vi "CurlingRobotforSweepFPGA.vi"() -> ()   [LabVIEW 2015]
uses:
  <vilib>/IEDriver/SPIandI2C/FPGA/Library/IP SPI&I2C.lvlib
  <vilib>/eio/EIONode/EIONode.xnode
  <vilib>/rvi/eio/common/nirviEmuTemplateMethod_errors.vi
  <vilib>/Platform/TimedLoop/XDataNode/wakeup.ctl
  <vilib>/Platform/TimedLoop/XDataNode/XDNodeRunTimeDep.lvlib
  <vilib>/Platform/TimedLoop/XDataNode/nitl_modes.ctl
  <vilib>/Platform/TimedLoop/XDataNode/timing_clust.ctl
  <vilib>/Platform/TimedLoop/XDataNode/XDataNode.xnode
  <vilib>/IEDriver/SPIandI2C/FPGA/Private/Initialize Port (I2C).vi
  <vilib>/IEDriver/SPIandI2C/FPGA/Private/IP Port (I2C).vi
  <vilib>/IEDriver/SPIandI2C/FPGA/Private/Configure Port (I2C).vi
  <vilib>/IEDriver/SPIandI2C/FPGA/Private/Arm Port (I2C).vi
  <vilib>/IEDriver/SPIandI2C/FPGA/Private/Write Port (I2C).vi
  <vilib>/IEDriver/SPIandI2C/FPGA/Private/Read Port (I2C).vi
panel:
  out "FPGA_I2C_port0":i32
  out "FPGA_I2C_port2":i32
  in  "I2C Protocol Action 2":T1(ring)=enum."Idle"
  in  "I2C Protocol Input Data 2":u8
  out "Write Done 2":bool
  out "Arm Done 2":bool
  out "I2C Protocol Output Data 2":u8
  out "Read Done 2":bool
  in  "I2C Protocol Configure 2":T2 {"Command (Write & Read)" items=["Write & Read", "Write", "Read"]}
  out "Configure Done 2":bool
  out "Steer_Left":i64=56
  in  "QuadENC2Reset 2":bool
  out "Steer_Right":i64=56
  in  "QuadENC3Reset 5":bool
  out "Steer_Rear":i64=56
  in  "QuadENC3Reset 4":bool
  in  "Steer_enable":fxp<+/-,20,5>
  in  "Drive_enable":fxp<+/-,20,5>
  in  "Elmo6_Steer_Rear":fxp<+/-,20,5>
  in  "Elmo5_Steer_Right":fxp<+/-,20,5>
  in  "Elmo4_Steer_Left":fxp<+/-,20,5>
  out "Driving_Rear":i64=56
  in  "QuadENC3Reset 3":bool
  in  "stop 2":bool
  in  "Elmo1_Left":fxp<+/-,20,5>
  in  "Elmo2_Right":fxp<+/-,20,5>
  in  "Elmo3_Rear":fxp<+/-,20,5>
  in  "stop":bool
  out "Driving_Left":i64=56
  in  "QuadENC2Reset":bool
  out "Driving_Right":i64=56
  in  "QuadENC3Reset 2":bool
  in  "I2C Protocol Action 0":T1(ring)=enum."Idle"
  in  "I2C Protocol Input Data 0":u8
  out "Write Done":bool
  out "Arm Done":bool
  out "I2C Protocol Output Data 0":u8
  out "Read Done":bool
  in  "I2C Protocol Configure 0":T2 {"Command (Write & Read)" items=["Write & Read", "Write", "Read"]}
  out "Configure Done":bool
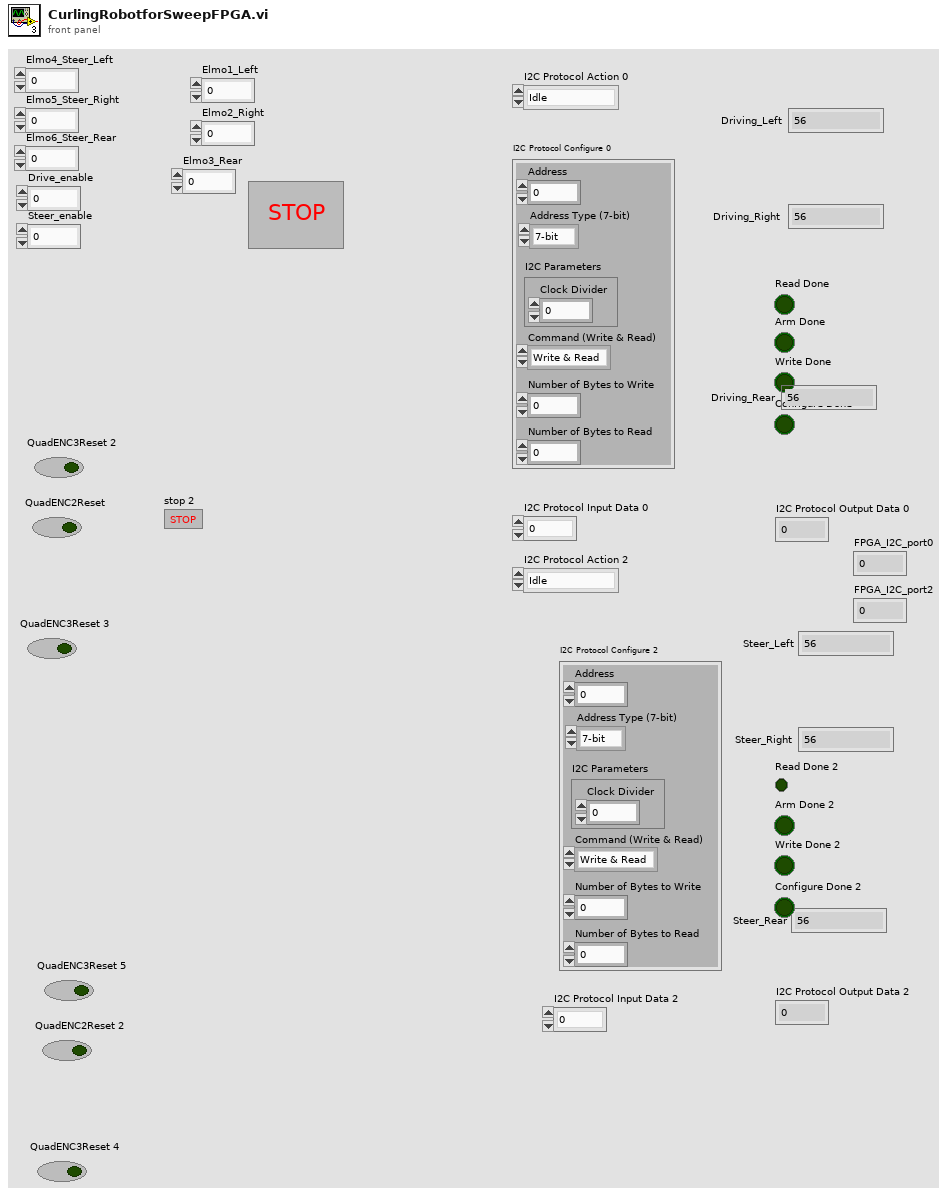
[diagram p1: front panel]
types:
  T1 = enum8{"Configure", "Write", "Arm", "Read", "Set Idle", "Idle"}
  T2 = cluster{"Address":u16, "Address Type (7-bit)":enum16{"7-bit", "10-bit"}, "I2C Parameters":cluster{"Clock Divider":u32}, "Command (Write & Read)":u8, "Number of Bytes to Write":u16, "Number of Bytes to Read":u16}
  T3 = typedef "IP SPI&I2C.lvlib/Private Data (I2C).ctl" = cluster{"Arm Trigger":refnum<k21>, "API to IP Data":refnum<k21>, "IP to API Data":refnum<k21>, "Configuration Register":refnum<k21>, "Configuration Lock":refnum<k21>}
  T4 = typedef "XDNodeRunTimeDep.lvlib/timing_clust.ctl" = cluster{"Expected End [f-1]":u64, "Actual End [f-1]":u64, "Finished Late? [f-1]":bool, "Expected End [i-1]":u64, "Actual End [i-1]":u64, "Finished Late? [i-1]":bool, "Expected Start [i]":u64, "Actual Start [i]":u64, "Expected Start [f]":u64, "Actual Start [f]":u64, "Source Name":string, "Structure Name":string, "Period":i64, "Deadline":i64, "Offset":i64, "Start":i64, "Priority":i32, "Timeout":i32, "Mode":T5, "Wakeup Reason":T6, "Error":errorcluster, "Source Type":string, "Secondary Source Type":string, "Global End Time":u64, "Global Start Time":u64, "Frame Duration":u64, "Iteration Duration":u64, "Assigned CPU":i32, "I/O Scan Engine Mode":u32}
  T5 = typedef "XDNodeRunTimeDep.lvlib/nitl_modes.ctl" = enum32{"No Change", "Process missed periods, maintain original phase", "Discard missed periods, maintain original phase", "Process missed periods, ignore original phase", "Discard missed periods, ignore original phase"}
  T6 = typedef "XDNodeRunTimeDep.lvlib/wakeup.ctl" = enum32{"Normal", "Aborted", "Asynchronous wakeup", "Timing source error", "Timed loop error", "Timeout"}
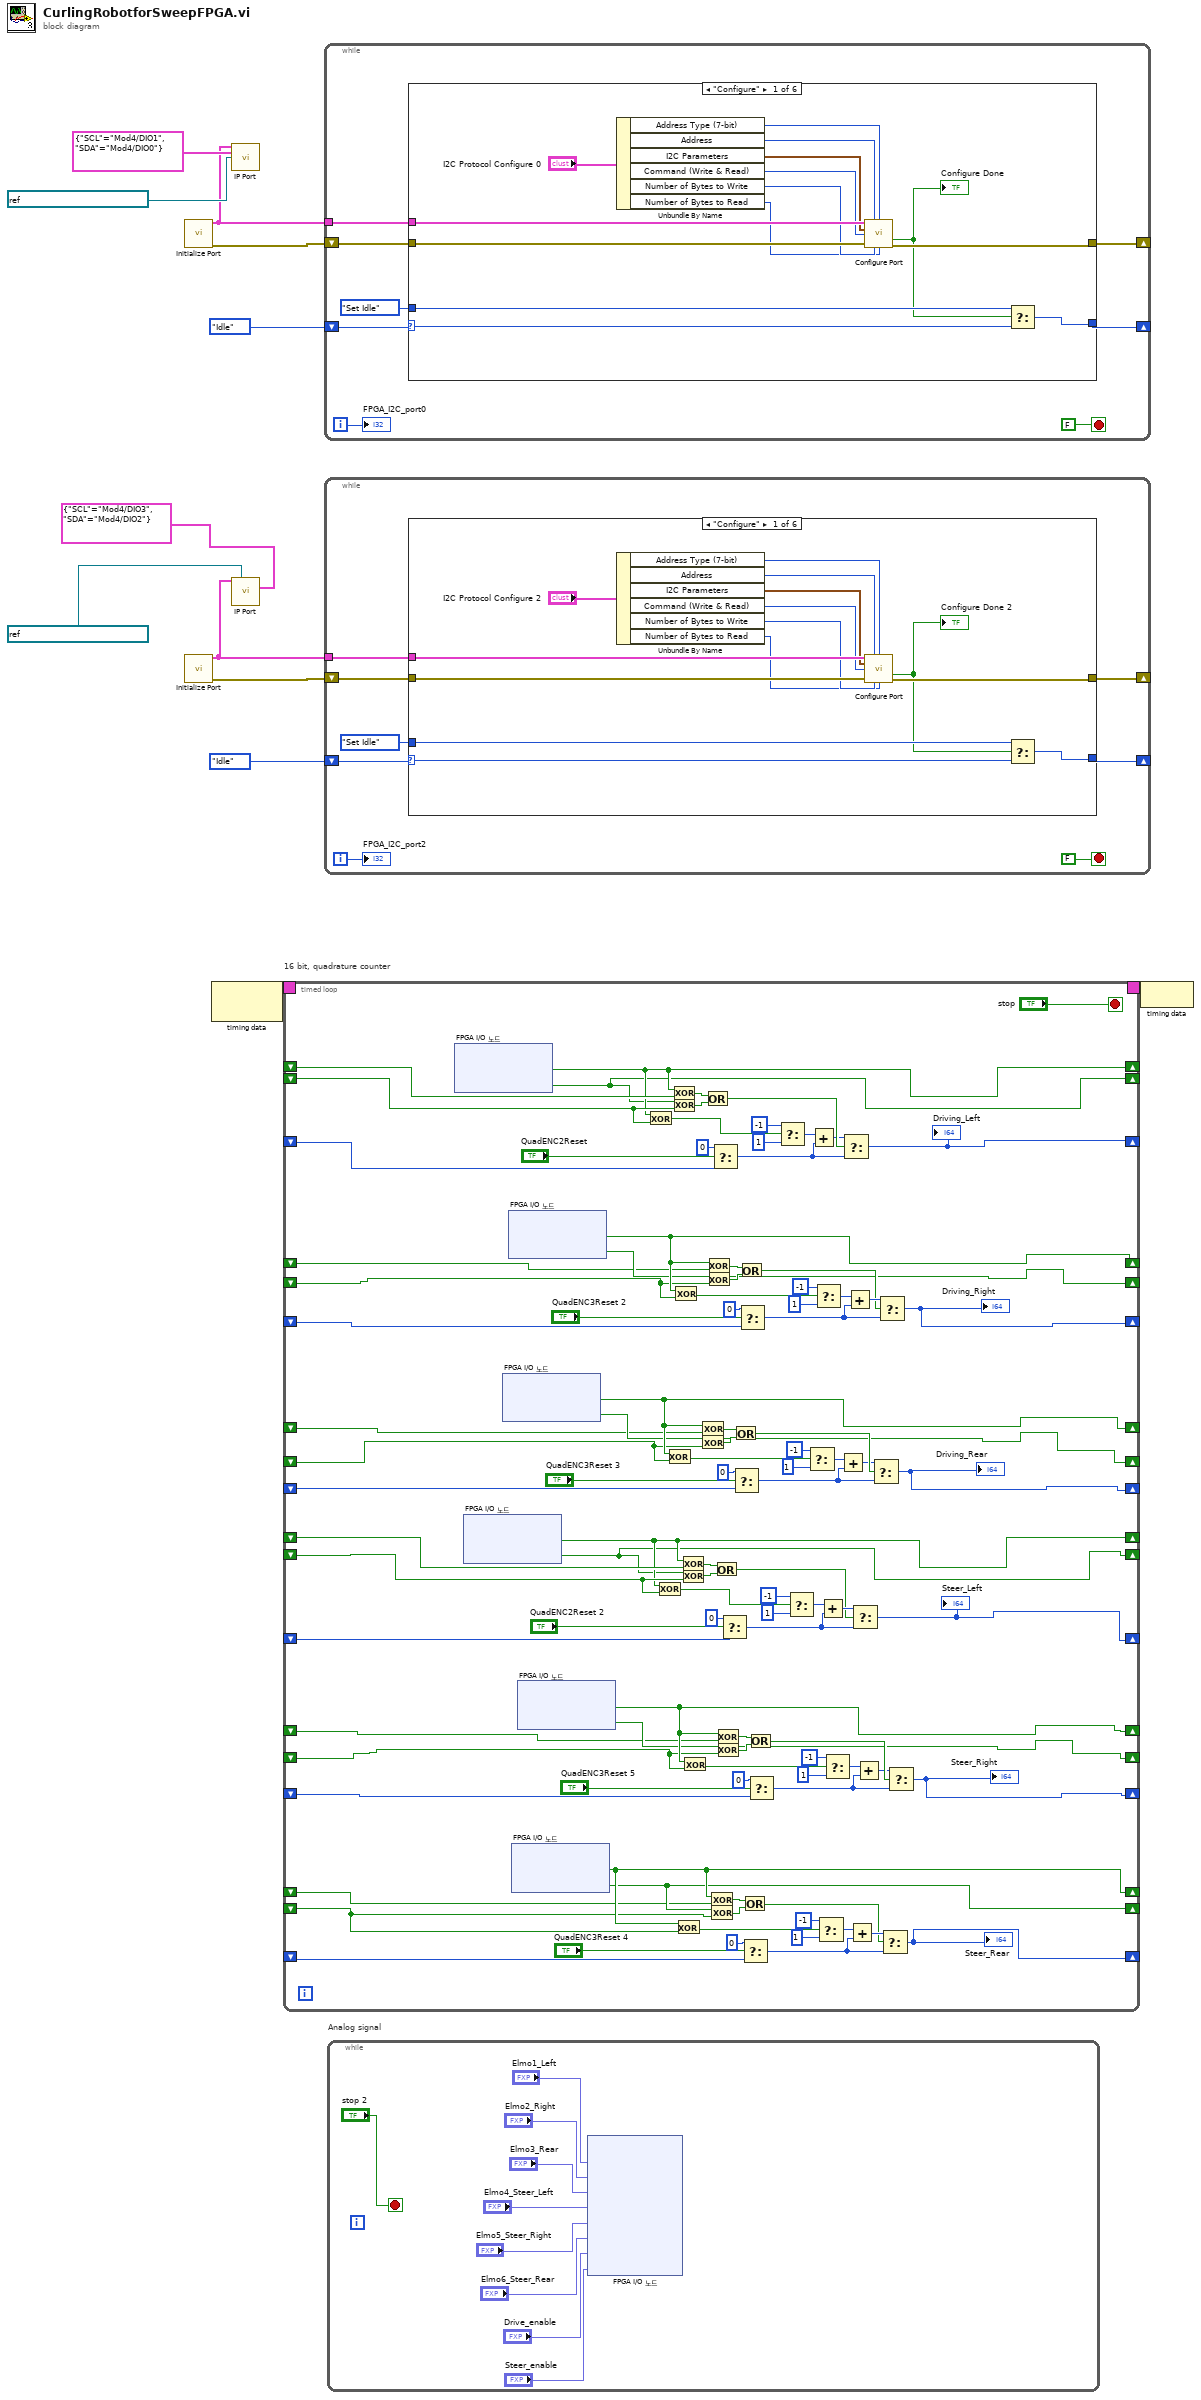
[diagram p0: block diagram]
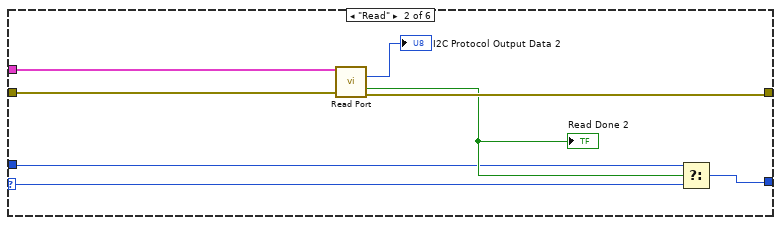
[diagram p2: hidden frame]
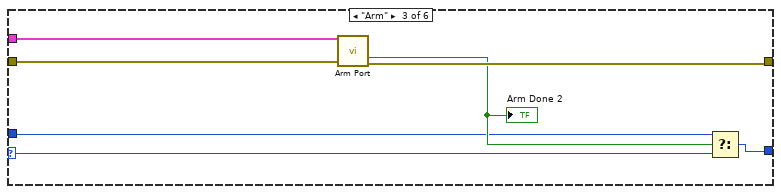
[diagram p3: hidden frame]
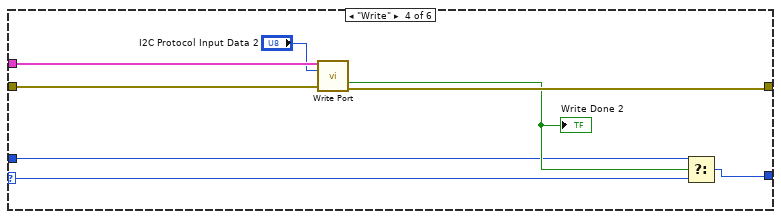
[diagram p4: hidden frame]
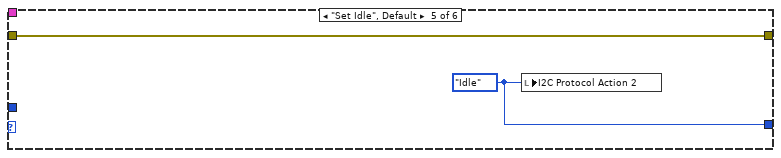
[diagram p5: hidden frame]
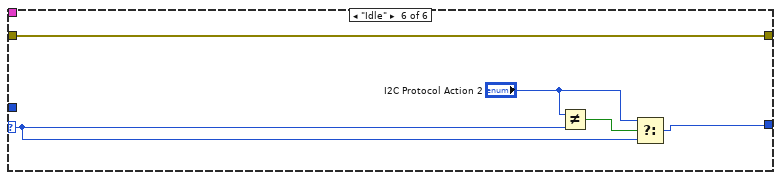
[diagram p6: hidden frame]
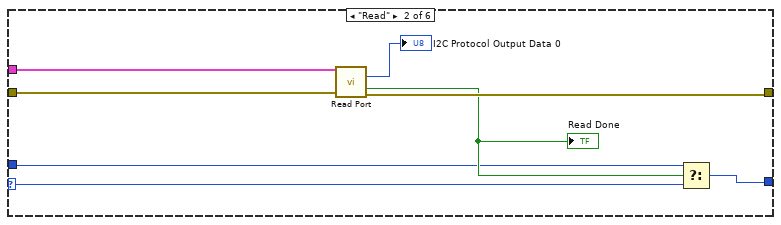
[diagram p7: hidden frame]
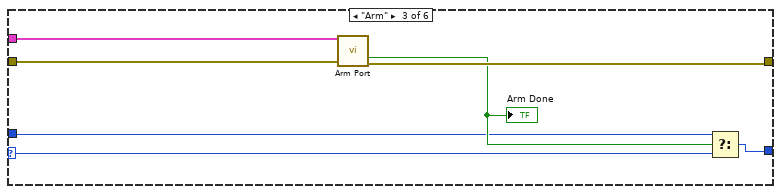
[diagram p8: hidden frame]
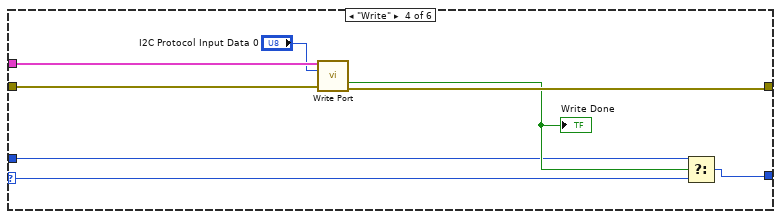
[diagram p9: hidden frame]
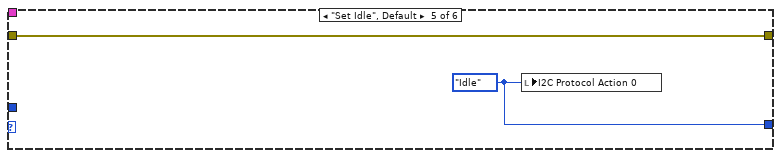
[diagram p10: hidden frame]
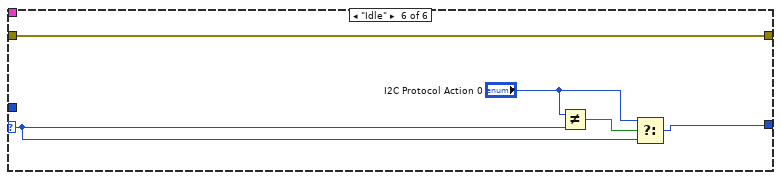
[diagram p11: hidden frame]
diagram:
  n1 = call-poly <vilib>:"Initialize Port.vi"() -> ("Private Data Out"=w8:T3, "error out"=w7:errorcluster)  [unwired: 14 in]
  n2 = call-poly <vilib>:"Initialize Port.vi"() -> ("Private Data Out"=w3:T3, "error out"=w4:errorcluster)  [unwired: 14 in]
  n3 = node-c288() -> (w12:T4)  [unwired: 1 in]
  n4 = call-poly <vilib>:"IP Port.vi"("Private Data In"=w8, "I2C FPGA IO"=cluster{"SCL":refnum<k21>, "SDA":refnum<k21>} {"SCL"="Mod4/DIO1", "SDA"="Mod4/DIO0"}, "FPGA Clock"=refnum<k21> "40 MHz Onboard Clock") -> ()  [unwired: 13 in]
  n5 = call-poly <vilib>:"IP Port.vi"("Private Data In"=w3, "I2C FPGA IO"=cluster{"SCL":refnum<k21>, "SDA":refnum<k21>} {"SCL"="Mod4/DIO3", "SDA"="Mod4/DIO2"}, "FPGA Clock"=refnum<k21> "40 MHz Onboard Clock") -> ()  [unwired: 13 in]
  n6 = timed-loop "16 bit, quadrature counter" {
    shift-left: _ -> [w102]
    shift-right: [w100] -> _
    shift-left: _ -> [w103]
    shift-right: [w101] -> _
    shift-right: [w82] -> _
    shift-left: _ -> [w99]
    timing: w12 -> [_]
    timing-out: [_] -> w11
    shift-right: [w87] -> _
    shift-left: _ -> [w85]
    shift-right: [w86] -> _
    shift-left: _ -> [w84]
    shift-right: [w13] -> _
    shift-left: _ -> [w83]
    shift-right: [w70] -> _
    shift-left: _ -> [w67]
    shift-right: [w69] -> _
    shift-left: _ -> [w66]
    shift-right: [w68] -> _
    shift-left: _ -> [w65]
    shift-right: [w28] -> _
    shift-left: _ -> [w31]
    shift-right: [w27] -> _
    shift-left: _ -> [w30]
    shift-right: [w26] -> _
    shift-left: _ -> [w29]
    shift-right: [w25] -> _
    shift-left: _ -> [w20]
    shift-right: [w24] -> _
    shift-left: _ -> [w21]
    shift-right: [w23] -> _
    shift-left: _ -> [w22]
    shift-right: [w19] -> _
    shift-left: _ -> [w15]
    shift-right: [w18] -> _
    shift-left: _ -> [w16]
    shift-right: [w17] -> _
    shift-left: _ -> [w14]
    stop <- "stop" stop-if-true
    n7 = xnode "FPGA I/O 노드"() -> ("Mod2/DIO1"=w101:bool, "Mod2/DIO2"=w100:bool)  [unwired: 2 in, 2 out]
    n8 = xnode "FPGA I/O 노드"() -> ("Mod3/DIO1"=w28:bool, "Mod3/DIO2"=w27:bool)  [unwired: 2 in, 2 out]
    n9 = xnode "FPGA I/O 노드"() -> ("Mod2/DIO5"=w70:bool, "Mod2/DIO6"=w69:bool)  [unwired: 2 in, 2 out]
    n10 = xnode "FPGA I/O 노드"() -> ("Mod2/DIO3"=w87:bool, "Mod2/DIO4"=w86:bool)  [unwired: 2 in, 2 out]
    n11 = xnode "FPGA I/O 노드"() -> ("Mod3/DIO5"=w19:bool, "Mod3/DIO6"=w18:bool)  [unwired: 2 in, 2 out]
    n12 = xnode "FPGA I/O 노드"() -> ("Mod3/DIO3"=w25:bool, "Mod3/DIO4"=w24:bool)  [unwired: 2 in, 2 out]
    n13 = Exclusive Or(1:w102, 2:w101) -> (0:w114:bool)
    n14 = Exclusive Or(1:w30, 2:w28) -> (0:w32:bool)
    n15 = Exclusive Or(1:w66, 2:w70) -> (0:w81:bool)
    n16 = Exclusive Or(1:w103, 2:w101) -> (0:w112:bool)
    n17 = Exclusive Or(1:w102, 2:w100) -> (0:w111:bool)
    n18 = Exclusive Or(1:w84, 2:w87) -> (0:w88:bool)
    n19 = Exclusive Or(1:w16, 2:w19) -> (0:w54:bool)
    n20 = Exclusive Or(1:w31, 2:w28) -> (0:w34:bool)
    n21 = Exclusive Or(1:w30, 2:w27) -> (0:w35:bool)
    n22 = Exclusive Or(1:w21, 2:w25) -> (0:w53:bool)
    n23 = Exclusive Or(1:w67, 2:w70) -> (0:w79:bool)
    n24 = Exclusive Or(1:w66, 2:w69) -> (0:w78:bool)
    n25 = Or(x=w112, y=w111) -> (x .or. y?=w113:bool)
    n26 = Exclusive Or(1:w85, 2:w87) -> (0:w90:bool)
    n27 = Exclusive Or(1:w84, 2:w86) -> (0:w91:bool)
    n28 = Exclusive Or(1:w15, 2:w19) -> (0:w56:bool)
    n29 = Exclusive Or(1:w16, 2:w18) -> (0:w57:bool)
    n30 = Select(t=i64 0 ("16 bit"), s="QuadENC2Reset", f=w99) -> (s? t:f=w104:i64)
    n31 = Or(x=w34, y=w35) -> (x .or. y?=w33:bool)
    n32 = Exclusive Or(1:w20, 2:w25) -> (0:w51:bool)
    n33 = Exclusive Or(1:w21, 2:w24) -> (0:w50:bool)
    n34 = Select(t=i64 0 ("16 bit"), s="QuadENC2Reset 2", f=w29) -> (s? t:f=w42:i64)
    n35 = Or(x=w79, y=w78) -> (x .or. y?=w80:bool)
    n36 = Select(t=i64 0 ("16 bit"), s="QuadENC3Reset 3", f=w65) -> (s? t:f=w74:i64)
    n37 = Or(x=w90, y=w91) -> (x .or. y?=w89:bool)
    n38 = Select(t=i64 0 ("16 bit"), s="QuadENC3Reset 2", f=w83) -> (s? t:f=w95:i64)
    n39 = Or(x=w56, y=w57) -> (x .or. y?=w55:bool)
    n40 = Select(t=i64 0 ("16 bit"), s="QuadENC3Reset 4", f=w14) -> (s? t:f=w61:i64)
    n41 = Or(x=w51, y=w50) -> (x .or. y?=w52:bool)
    n42 = Select(t=i64 0 ("16 bit"), s="QuadENC3Reset 5", f=w22) -> (s? t:f=w46:i64)
    n43 = Select(t=i64 -1 ("16 bit"), s=w114, f=i64 1 ("16 bit")) -> (s? t:f=w108:i64)
    n44 = Select(t=i64 -1 ("16 bit"), s=w32, f=i64 1 ("16 bit")) -> (s? t:f=w38:i64)
    n45 = Select(t=i64 -1 ("16 bit"), s=w81, f=i64 1 ("16 bit")) -> (s? t:f=w75:i64)
    n46 = Add(x=w108, y=w104) -> (x+y=w106:i64)
    n47 = Select(t=i64 -1 ("16 bit"), s=w88, f=i64 1 ("16 bit")) -> (s? t:f=w94:i64)
    n48 = Select(t=i64 -1 ("16 bit"), s=w54, f=i64 1 ("16 bit")) -> (s? t:f=w60:i64)
    n49 = Add(x=w38, y=w42) -> (x+y=w40:i64)
    n50 = Select(t=i64 -1 ("16 bit"), s=w53, f=i64 1 ("16 bit")) -> (s? t:f=w47:i64)
    n51 = Add(x=w75, y=w74) -> (x+y=w72:i64)
    n52 = Select(t=w106, s=w113, f=w104) -> (s? t:f=w82:i64)
    "Driving_Left" <- w82
    n53 = Add(x=w94, y=w95) -> (x+y=w97:i64)
    n54 = Add(x=w60, y=w61) -> (x+y=w63:i64)
    n55 = Select(t=w40, s=w33, f=w42) -> (s? t:f=w26:i64)
    "Steer_Left" <- w26
    n56 = Add(x=w47, y=w46) -> (x+y=w44:i64)
    n57 = Select(t=w72, s=w80, f=w74) -> (s? t:f=w68:i64)
    "Driving_Rear" <- w68
    n58 = Select(t=w97, s=w89, f=w95) -> (s? t:f=w13:i64)
    "Driving_Right" <- w13
    n59 = Select(t=w63, s=w55, f=w61) -> (s? t:f=w17:i64)
    "Steer_Rear" <- w17
    n60 = Select(t=w44, s=w52, f=w46) -> (s? t:f=w23:i64)
    "Steer_Right" <- w23
  }
  n61 = while {
    shift-right: [w122] -> _
    shift-left: w7 -> [w124]
    tunnel: w8 -> [w125]
    shift-right: [w120] -> _
    shift-left: T1."Idle" ("Action") -> [w121]
    i -> [w118]
    stop <- FALSE stop-if-true
    n62 = case shown="\"Configure\"" w121 {
      selector: w121 -> [w130 w141 w149 w156 _ w166]
      tunnel: w125 -> [w139 w147 w154 w162 _ _]
      tunnel: w124 -> [w138 w146 w153 w161 w164 w169]
      tunnel: [w137 w145 w152 w160 w164 w169] -> w122
      tunnel: [w131 w143 w151 w157 w163 w165] -> w120
      tunnel: T1."Set Idle" ("Action") -> [w129 w140 w148 w155 _ _]
      frame "Configure" {
        n63 = Unbundle By Name("I2C Protocol Configure 0") -> ("Address Type (7-bit)"=w135:enum16{"7-bit", "10-bit"}, "Address"=w126:u16, "I2C Parameters"=w134:cluster{"Clock Divider":u32}, "Command (Write & Read)"=w127:u8, "Number of Bytes to Write"=w133:u16, "Number of Bytes to Read"=w132:u16)
        n64 = call-poly <vilib>:"Configure Port.vi"("Private Data In"=w139, "Address"=w126, "Address Type (7-bit)"=w135, "I2C Parameters"=w134, "Command (Write & Read)"=w127, "error in"=w138, "Number of Bytes to Write"=w133, "Number of Bytes to Read"=w132) -> ("Done"=w128:bool, "error out"=w137:errorcluster)  [unwired: 5 in, 1 out]
        "Configure Done" <- w128
        n65 = Select(t=w129, s=w128, f=w130) -> (s? t:f=w131:T1)
      }
      frame "Read" {
        n66 = call-poly <vilib>:"Read Port.vi"("Private Data In"=w147, "error in"=w146) -> ("Data Out"=→"I2C Protocol Output Data 0":u8, "Output Valid"=w142:bool, "error out"=w145:errorcluster)  [unwired: 10 in, 1 out]
        "Read Done" <- w142
        n67 = Select(t=w140, s=w142, f=w141) -> (s? t:f=w143:T1)
      }
      frame "Arm" {
        n68 = call-poly <vilib>:"Arm Port.vi"("Private Data In"=w154, "error in"=w153) -> ("Done"=w150:bool, "error out"=w152:errorcluster)  [unwired: 11 in, 1 out]
        "Arm Done" <- w150
        n69 = Select(t=w148, s=w150, f=w149) -> (s? t:f=w151:T1)
      }
      frame "Write" {
        n70 = call-poly <vilib>:"Write Port.vi"("Private Data In"=w162, "Data In"="I2C Protocol Input Data 0", "error in"=w161) -> ("Done"=w158:bool, "error out"=w160:errorcluster)  [unwired: 10 in, 1 out]
        "Write Done" <- w158
        n71 = Select(t=w155, s=w158, f=w156) -> (s? t:f=w157:T1)
      }
      frame "Set Idle", Default {
        w163 = T1."Idle" ("Action")
        n72 = local write "I2C Protocol Action 0"(w163) -> ()
      }
      frame "Idle" {
        n73 = Not Equal?(x="I2C Protocol Action 0", y=w166) -> (x != y?=w168:bool)
        n74 = Select(t="I2C Protocol Action 0", s=w168, f=w166) -> (s? t:f=w165:T1)
      }
    }
    "FPGA_I2C_port0" <- w118
  }
  n75 = while {
    shift-right: [w174] -> _
    shift-left: w4 -> [w176]
    tunnel: w3 -> [w177]
    shift-right: [w172] -> _
    shift-left: T1."Idle" ("Action") -> [w173]
    i -> [w170]
    stop <- FALSE stop-if-true
    n76 = case shown="\"Configure\"" w173 {
      selector: w173 -> [w182 w193 w201 w208 _ w218]
      tunnel: w177 -> [w191 w199 w206 w214 _ _]
      tunnel: w176 -> [w190 w198 w205 w213 w216 w221]
      tunnel: [w189 w197 w204 w212 w216 w221] -> w174
      tunnel: [w183 w195 w203 w209 w215 w217] -> w172
      tunnel: T1."Set Idle" ("Action") -> [w181 w192 w200 w207 _ _]
      frame "Configure" {
        n77 = Unbundle By Name("I2C Protocol Configure 2") -> ("Address Type (7-bit)"=w187:enum16{"7-bit", "10-bit"}, "Address"=w178:u16, "I2C Parameters"=w186:cluster{"Clock Divider":u32}, "Command (Write & Read)"=w179:u8, "Number of Bytes to Write"=w185:u16, "Number of Bytes to Read"=w184:u16)
        n78 = call-poly <vilib>:"Configure Port.vi"("Private Data In"=w191, "Address"=w178, "Address Type (7-bit)"=w187, "I2C Parameters"=w186, "Command (Write & Read)"=w179, "error in"=w190, "Number of Bytes to Write"=w185, "Number of Bytes to Read"=w184) -> ("Done"=w180:bool, "error out"=w189:errorcluster)  [unwired: 5 in, 1 out]
        "Configure Done 2" <- w180
        n79 = Select(t=w181, s=w180, f=w182) -> (s? t:f=w183:T1)
      }
      frame "Read" {
        n80 = call-poly <vilib>:"Read Port.vi"("Private Data In"=w199, "error in"=w198) -> ("Data Out"=→"I2C Protocol Output Data 2":u8, "Output Valid"=w194:bool, "error out"=w197:errorcluster)  [unwired: 10 in, 1 out]
        "Read Done 2" <- w194
        n81 = Select(t=w192, s=w194, f=w193) -> (s? t:f=w195:T1)
      }
      frame "Arm" {
        n82 = call-poly <vilib>:"Arm Port.vi"("Private Data In"=w206, "error in"=w205) -> ("Done"=w202:bool, "error out"=w204:errorcluster)  [unwired: 11 in, 1 out]
        "Arm Done 2" <- w202
        n83 = Select(t=w200, s=w202, f=w201) -> (s? t:f=w203:T1)
      }
      frame "Write" {
        n84 = call-poly <vilib>:"Write Port.vi"("Private Data In"=w214, "Data In"="I2C Protocol Input Data 2", "error in"=w213) -> ("Done"=w210:bool, "error out"=w212:errorcluster)  [unwired: 10 in, 1 out]
        "Write Done 2" <- w210
        n85 = Select(t=w207, s=w210, f=w208) -> (s? t:f=w209:T1)
      }
      frame "Set Idle", Default {
        w215 = T1."Idle" ("Action")
        n86 = local write "I2C Protocol Action 2"(w215) -> ()
      }
      frame "Idle" {
        n87 = Not Equal?(x="I2C Protocol Action 2", y=w218) -> (x != y?=w220:bool)
        n88 = Select(t="I2C Protocol Action 2", s=w220, f=w218) -> (s? t:f=w217:T1)
      }
    }
    "FPGA_I2C_port2" <- w170
  }
  n89 = while "Analog signal" {
    stop <- "stop 2" stop-if-true
    n90 = xnode "FPGA I/O 노드"("Mod1/AO0"="Elmo1_Left", "Mod1/AO1"="Elmo2_Right", "Mod1/AO2"="Elmo3_Rear", "Mod1/AO3"="Elmo4_Steer_Left", "Mod1/AO4"="Elmo5_Steer_Right", "Mod1/AO5"="Elmo6_Steer_Rear", "Mod1/AO6"="Drive_enable", "Mod1/AO7"="Steer_enable") -> ()  [unwired: 8 in, 8 out]
  }
  n91 = node-c288(w11) -> ()
